vi "correlation_X.vi"(11 "传递变量":T1) -> (3 "数值":i32)   [LabVIEW 2013]
uses:
  <vilib>/Analysis/2dsp.llb/1D Cross Correlation (DBL).vi
  <vilib>/Analysis/NI_AALPro.lvlib
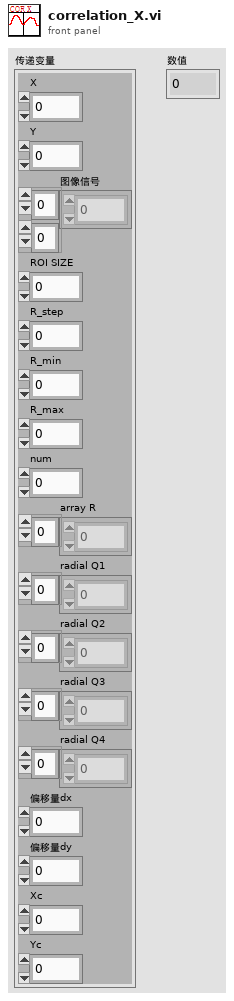
[diagram p1: front panel]
types:
  T1 = cluster{"X":dbl, "Y":dbl, "图像信号":dbl[][], "ROI SIZE":i32, "R_step":dbl, "R_min":dbl, "R_max":dbl, "num":dbl, "array R":dbl[], "radial Q1":dbl[], "radial Q2":dbl[], "radial Q3":dbl[], "radial Q4":dbl[], "偏移量dx":dbl, "偏移量dy":dbl, "Xc":dbl, "Yc":dbl}
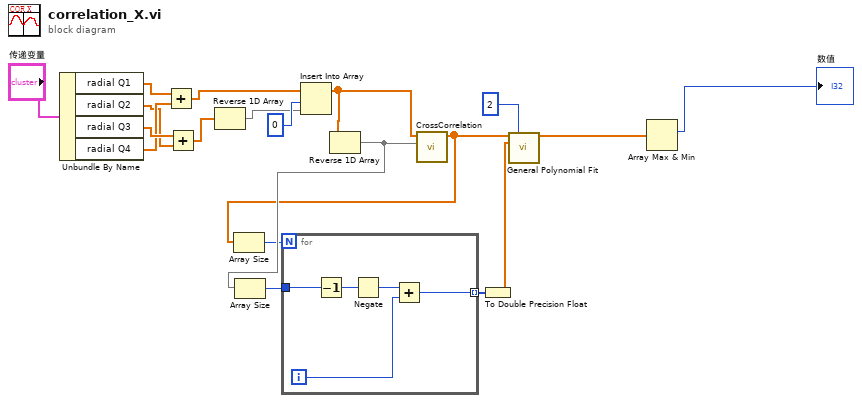
[diagram p0: block diagram]
diagram:
  n1 = Unbundle By Name("传递变量") -> ("radial Q1"=w5:dbl[], "radial Q2"=w1:dbl[], "radial Q3"=w4:dbl[], "radial Q4"=w2:dbl[])
  n2 = Add(x=w5, y=w2) -> (x+y=w3:dbl[])
  n3 = Add(x=w4, y=w1) -> (x+y=w6:dbl[])
  n4 = Reverse 1D Array(array=w6) -> (reversed array=w7:dbl[])
  n5 = Insert Into Array(array=w3, index=0 ("索引"), new element=w7) -> (w9:dbl[])
  n6 = Reverse 1D Array(array=w9) -> (reversed array=w12:dbl[])
  n7 = Array Size(array=w12) -> (size(s)=w13:i32)
  n8 = call-poly <vilib>:"CrossCorrelation.vi"("Y"=w12, "X"=w9) -> ("Rxy"=w10:dbl[])  [unwired: 8 in, 1 out]
  n9 = Array Size(array=w10) -> (size(s)=w11:i32)
  n10 = for {
    N: w11 -> [_]
    tunnel: w13 -> [w22]
    tunnel: [w20] -> w14 mode=indexing
    i -> [w21]
    n11 = Decrement(x=w22) -> (x-1=w24:i32)
    n12 = Negate(x=w24) -> (-x=w23:i32)
    n13 = Add(x=w23, y=w21) -> (x+y=w20:i32)
  }
  n14 = To Double Precision Float(number=w14) -> (double precision float=w15:dbl[])
  n15 = call <vilib>:"General Polynomial Fit.vi"("Y"=w10, "polynomial order"=2, "X"=w15) -> ("Best Polynomial Fit"=w17:dbl[])  [unwired: 9 in, 3 out]
  n16 = Array Max & Min(array=w17) -> (max index (indices)=→"数值":i32)  [unwired: 3 out]
